vi "Get gRPC ID.vi"(11 "OOP Server in":refnum<class "OOP Server.lvclass">) -> (2 "gRPC ID":T1, 3 "OOP Server out":refnum<class "OOP Server.lvclass">)   [LabVIEW 2019, in "OOP Server.lvlib" / "OOP Server.lvclass"]
uses:
  OOP Server.lvclass
  gRPC interface/Server API/typeDefs/grpcId.ctl
  OOP Server.lvclass/OOP Server.ctl
  gRPC interface/gprc-lvsupport.lvlib
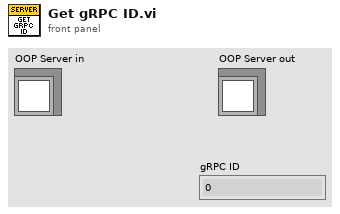
[diagram p1: front panel]
types:
  T1 = typedef "gprc-lvsupport.lvlib/grpcId.ctl" = u64
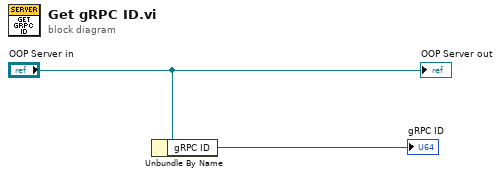
[diagram p0: block diagram]
diagram:
  n1 = Unbundle By Name("OOP Server in") -> ("gRPC ID"=→"gRPC ID":T1)
  "OOP Server out" <- "OOP Server in"
